vi "Read Data.vi"(8 "error in (no error)":errorcluster, 11 "Neocera LTC-21 in":refnum<class "Neocera LTC-21.lvclass">) -> (0 "error out":errorcluster, 2 "Data":waveform(dbl)[](array[waveform]), 3 "Neocera LTC-21 out":refnum<class "Neocera LTC-21.lvclass">)   [LabVIEW 2015, in "Neocera LTC-21.lvclass"]
uses:
  Neocera LTC-21.lvclass
  Neocera Front Panel Data.ctl
  Neocera Heater Ranges.ctl
  Neocera Set Point Aproach.ctl
  OO Devices/Device/Read Control Panel Loaded.vi
  Instrument/Read VISA Resource.vi
  OO Devices/Device/Read Controls Snapshot.vi
  Instrument/Write VISA Resource.vi
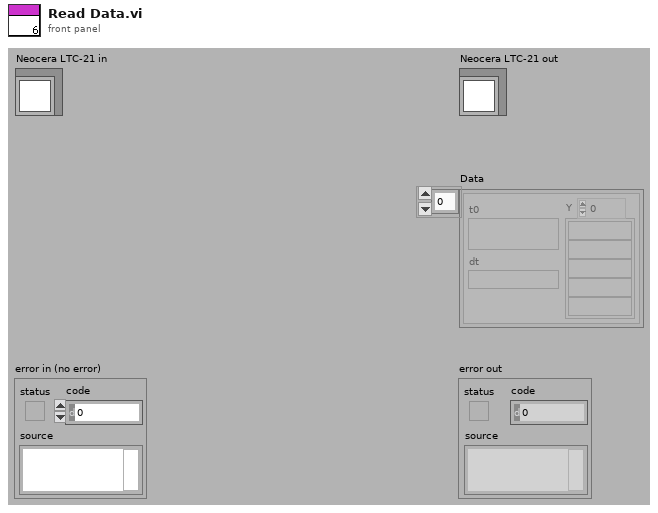
[diagram p1: front panel]
types:
  T1 = typedef "Neocera Front Panel Data.ctl" = cluster{"Channels to measure":dbl[], "Record heater":bool, "Set point":dbl, "Set Heater Range":T2, "Control":bool, "Approach":T3, "Ramp rate, K/min":dbl, "Control Channel":i16, "P":dbl, "I":dbl, "D":dbl, "Suspend heater":bool}
  T2 = typedef "Neocera Heater Ranges.ctl" = enum16{"Off", "0.05W", "0.5W", "5W", "50W"}
  T3 = typedef "Neocera Set Point Aproach.ctl" = enum16{"Instant", "Ramp"}
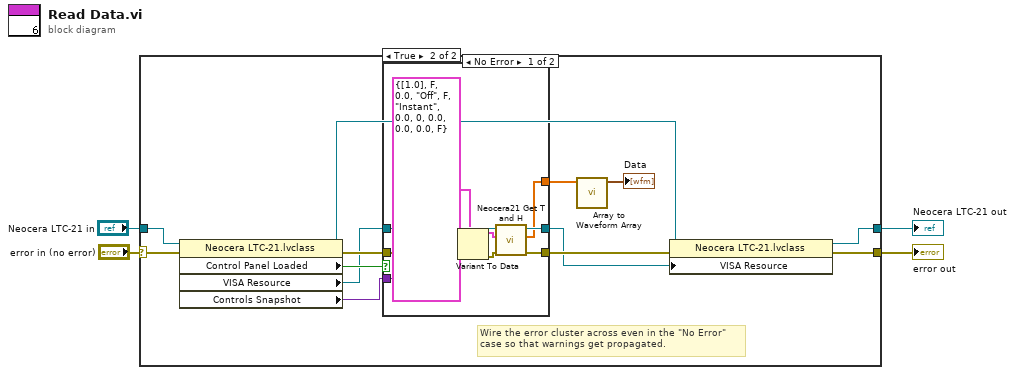
[diagram p0: block diagram]
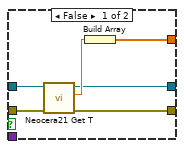
[diagram p2: hidden frame]
diagram:
  n1 = case shown="No Error" "error in (no error)" {
    selector: "error in (no error)" -> [w9 w34]
    tunnel: [w15 w34] -> w3
    tunnel: [w17 w33] -> w1
    tunnel: "Neocera LTC-21 in" -> [w8 w33]
    frame No Error {
      # "Wire the error cluster across even in the \"No Error\"\ncase so that warnings get propagated."
      n2 = property class="Neocera LTC-21.lvclass"(reference=w8, error in=w9) -> (reference out=w5:refnum<class "Neocera LTC-21.lvclass">, error out=w12:errorcluster, "Control Panel Loaded"=w11:bool, "VISA Resource"=w10:refnum<visa-resource-name>, "Controls Snapshot"=w6:variant)
      n3 = case shown="True" w11 {
        tunnel: [w18 w32] -> w7
        tunnel: [w23 w31] -> w16
        tunnel: w10 -> [w21 w30]
        tunnel: [w19 w29] -> w13
        tunnel: w12 -> [w22 w24]
        tunnel: w6 -> [_ w25]
        frame False {
          n4 = call "Neocera21 Get T.vi"("error in (no error)"=w22, "VISA Resource Name"=w21) -> ("error out"=w23:errorcluster, "Temperature"=w20:dbl, "VISA Resource Name Out"=w18:refnum<visa-resource-name>)  [unwired: 6 in, 1 out]
          n5 = Build Array(w20) -> (w19:dbl[])
        }
        frame True {
          n6 = Variant To Data(error in=w24, type=T1 {"Channels to measure"=[1.0], "Record heater"=FALSE, "Set point"=0.0, "Set Heater Range"=enum."Off", "Control"=FALSE, "Approach"=enum."Instant", "Ramp rate, K/min"=0.0, "Control Channel"=0, "P"=0.0, "I"=0.0, "D"=0.0, "Suspend heater"=FALSE} ("Private data"), Variant=w25) -> (data=w27:T1, error out=w26:errorcluster)
          n7 = call "Neocera21 Get T and H.vi"("error in (no error)"=w26, "Private data"=w27, "VISA Resource Name"=w30) -> ("error out"=w31:errorcluster, "Data out"=w29:dbl[], "VISA Resource Name Out"=w32:refnum<visa-resource-name>)  [unwired: 4 in, 2 out]
        }
      }
      n8 = call "Array to Waveform Array.vi"("Array"=w13) -> ("Waveform"=→"Data":waveform(dbl)[])  [unwired: 10 in]
      n9 = property class="Neocera LTC-21.lvclass"(reference=w5, error in=w16, "VISA Resource"=w7) -> (reference out=w17:refnum<class "Neocera LTC-21.lvclass">, error out=w15:errorcluster)
    }
    frame Error {
    }
  }
  "error out" <- w3
  "Neocera LTC-21 out" <- w1
